vi "Gyro.vi"   [LabVIEW 2016]
uses:
  CRC32/CRC32Settings.ctl
  DIOSerialPort/DIOSerialPortSettings.ctl
types:
  T1 = typedef "DIOSerialPortSettings.ctl" = cluster{"TxPort":refnum<k21>, "TxDataFIFO":refnum<k21>, "RxPort":refnum<k21>, "RxDataFIFO":refnum<k21>}
  T2 = typedef "CRC32Settings.ctl" = cluster{"DataFIFO":refnum<k21>, "CalculateFIFO":refnum<k21>, "CRCFIFO":refnum<k21>}
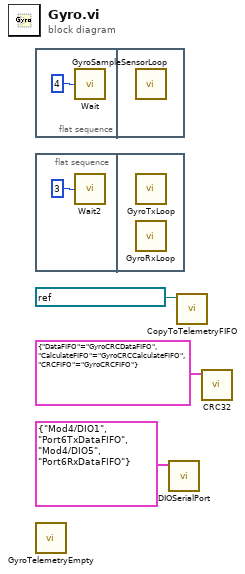
[diagram p0: block diagram]
diagram:
  n1 = flat-sequence {
    frame #0 {
      n2 = call "Wait"("Count(mSec)"=u8 4) -> ()  [unwired: 1 out]
    }
    frame #1 {
      n3 = call "GyroSampleSensorLoop.vi"() -> ()  [unwired: 12 in]
    }
  }
  n4 = flat-sequence {
    frame #0 {
      n5 = call "Wait2"("Count(mSec)"=u8 3) -> ()  [unwired: 1 out]
    }
    frame #1 {
      n6 = call "GyroTxLoop.vi"() -> ()  [unwired: 12 in]
      n7 = call "GyroRxLoop.vi"() -> ()  [unwired: 12 in]
    }
  }
  n8 = call "GyroTelemetryEmpty.vi"() -> ()  [unwired: 12 in]
  n9 = call "DIOSerialPort.vi"("DIOSerialPortSettings"=T1 {"TxPort"="Mod4/DIO1", "TxDataFIFO"="Port6TxDataFIFO", "RxPort"="Mod4/DIO5", "RxDataFIFO"="Port6RxDataFIFO"}) -> ()  [unwired: 11 in]
  n10 = call "CopyToTelemetryFIFO.vi"("SourceFIFO"=refnum<k21> "GyroTelemetryFIFO") -> ()  [unwired: 11 in]
  n11 = call "CRC32.vi"("CRC32Settings"=T2 {"DataFIFO"="GyroCRCDataFIFO", "CalculateFIFO"="GyroCRCCalculateFIFO", "CRCFIFO"="GyroCRCFIFO"}) -> ()  [unwired: 11 in]
